vi "Sperre telebuf Minerva 27 Bytes (Sub VI).vi"(0 "Thruster rpms":dbl[](array[numeric]), 1 "manip1":u8, 2 "manip2":u8, 3 "manip3":u8, 4 "Pan_tilt":bool[](array[boolean]), 5 "error in":errorcluster, 6 "dim 1+2":u8, 7 "Lights_HMI":bool[](array[boolean]), 8 "dim 3+4":u8, 9 "Zoom":bool[](array[boolean]), 11 "Power":bool[](array[boolean]), 12 "camera":u8=2) -> (14 "telebuf":u8[](array[numeric]), 19 "error IO":errorcluster)   [LabVIEW 2014]
uses:
  <vilib>/imath/engines/lvmath2/RunTimeEngine/BuiltInFunctions/uint8/NIMS_uint8(int).vi
  <instcachedir>/0/NIMS_uint8(int)_9D6EF81F86254677BB00410F9E5C6A1D.lvgen/NIMS_uint8(int)_9D6EF81F86254677BB00410F9E5C6A1D_001.vi
  <vilib>/imath/engines/lvmath2/RunTimeEngine/BuiltInFunctions/round/NIMS_round(DBL-S).vi
  <vilib>/imath/engines/lvmath2/RunTimeEngine/BuiltInFunctions/uint8/NIMS_uint8(real).vi
  <instcachedir>/0/NIMS_uint8(real)_CAA419FBB1354DA296C59E18C46DECF0.lvgen/NIMS_uint8(real)_CAA419FBB1354DA296C59E18C46DECF0_000.vi
  <instcachedir>/0/NIMS_uint8(int)_9D6EF81F86254677BB00410F9E5C6A1D.lvgen/NIMS_uint8(int)_9D6EF81F86254677BB00410F9E5C6A1D_000.vi
  <vilib>/imath/engines/lvmath2/RunTimeEngine/IndexReplace/NIMS V(S)=S.vi
  <instcachedir>/0/NIMS V(S)=S_2D52C4EC15D8415E870AEE69FB516CCA.lvgen/NIMS V(S)=S_2D52C4EC15D8415E870AEE69FB516CCA_005.vi
  <vilib>/imathl/engines/lvmath/Functions/Error Handling/Create Error.vi
  <vilib>/imath/engines/lvmath2/RunTimeEngine/BuiltInFunctions/bitand/NIMS_bitand(SorS,SorS).vi
  <instcachedir>/0/NIMS V(S)=S_2D52C4EC15D8415E870AEE69FB516CCA.lvgen/NIMS V(S)=S_2D52C4EC15D8415E870AEE69FB516CCA_000.vi
  <vilib>/imath/engines/lvmath2/RunTimeEngine/ErrorHandling/NIMS_Create Error From Enums.vi
  <vilib>/imath/engines/lvmath2/RunTimeEngine/IndexRead/NIMS V(S).vi
  <instcachedir>/0/NIMS V(S)_0488751826AF41519A22953C041130DC.lvgen/NIMS V(S)_0488751826AF41519A22953C041130DC_000.vi
  <vilib>/imath/engines/lvmath2/RunTimeEngine/BuiltInFunctions/bitset/NIMS_bitset(RS,RS,RS).vi
  <vilib>/imath/engines/lvmath2/RunTimeEngine/BuiltInFunctions/bitget/NIMS_bitget(SorS,SorS).vi
  <vilib>/imath/engines/lvmath2/RunTimeEngine/RangeToken/NIMS_Range_R2 - Integer.vi
  <instcachedir>/0/NIMS_Range_R2 - Integer_2D1304BAF97744E0A293025746CBADFC.lvgen/NIMS_Range_R2 - Integer_2D1304BAF97744E0A293025746CBADFC_000.vi
  <vilib>/imath/engines/lvmath2/RunTimeEngine/CommandStatement/MC_CommandStatement_break.vi
  <vilib>/imath/engines/lvmath2/RunTimeEngine/BuiltInFunctions/double/NIMS_double.vi
  <instcachedir>/0/NIMS_double_34E32F64C2B04A25A042F4CA881A0A41.lvgen/NIMS_double_34E32F64C2B04A25A042F4CA881A0A41_002.vi
  <vilib>/imath/engines/lvmath2/RunTimeEngine/BuiltInFunctions/mod/NIMS_mod_no_size_check.vi
  <instcachedir>/0/NIMS_mod_no_size_check_5393E3382FD241D281EEB71DA286C65B.lvgen/NIMS_mod_no_size_check_5393E3382FD241D281EEB71DA286C65B_001.vi
  <vilib>/imath/engines/lvmath2/RunTimeEngine/NodeEndStatement/NIMS_NodeEndStatement_Output.vi
  <instcachedir>/0/NIMS_NodeEndStatement_Output_53EC0D466D134D7ABD903AC30B43404B.lvgen/NIMS_NodeEndStatement_Output_53EC0D466D134D7ABD903AC30B43404B_017.vi
  <vilib>/imath/engines/lvmath2/RunTimeEngine/ErrorHandling/NIMS_Finalize Error.vi
panel:
  in  "UHI camera":bool=TRUE
  in  "Turbo":bool=TRUE
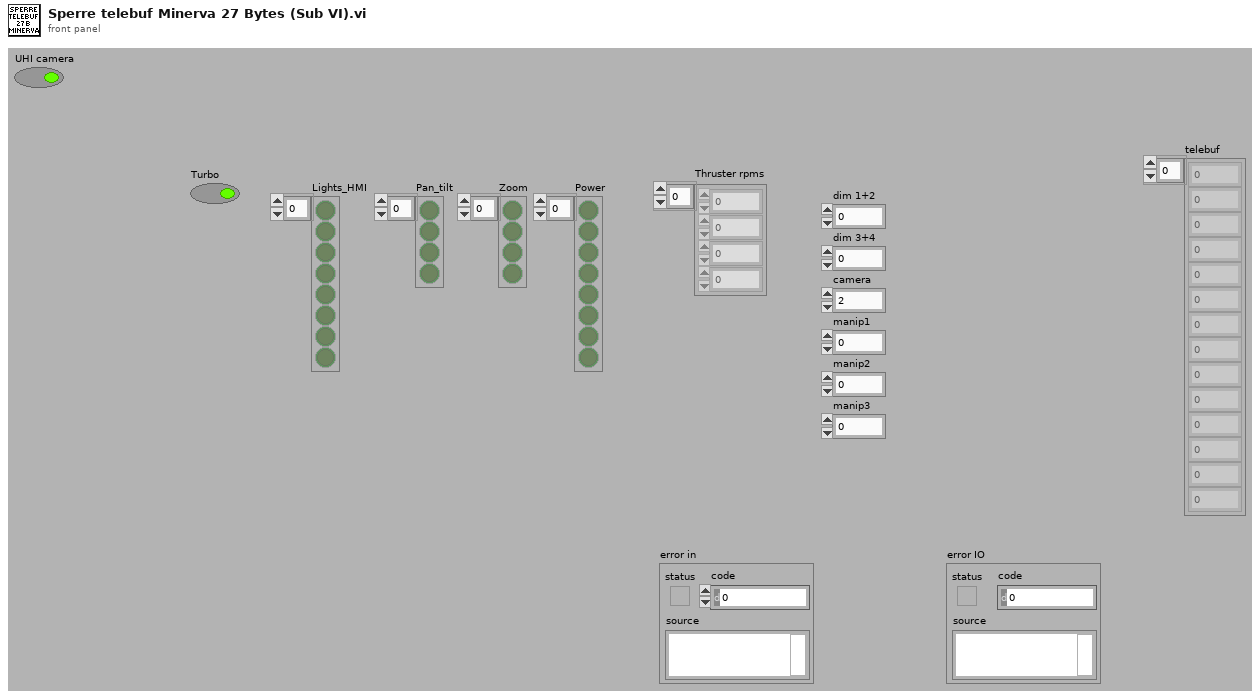
[diagram p1: front panel]
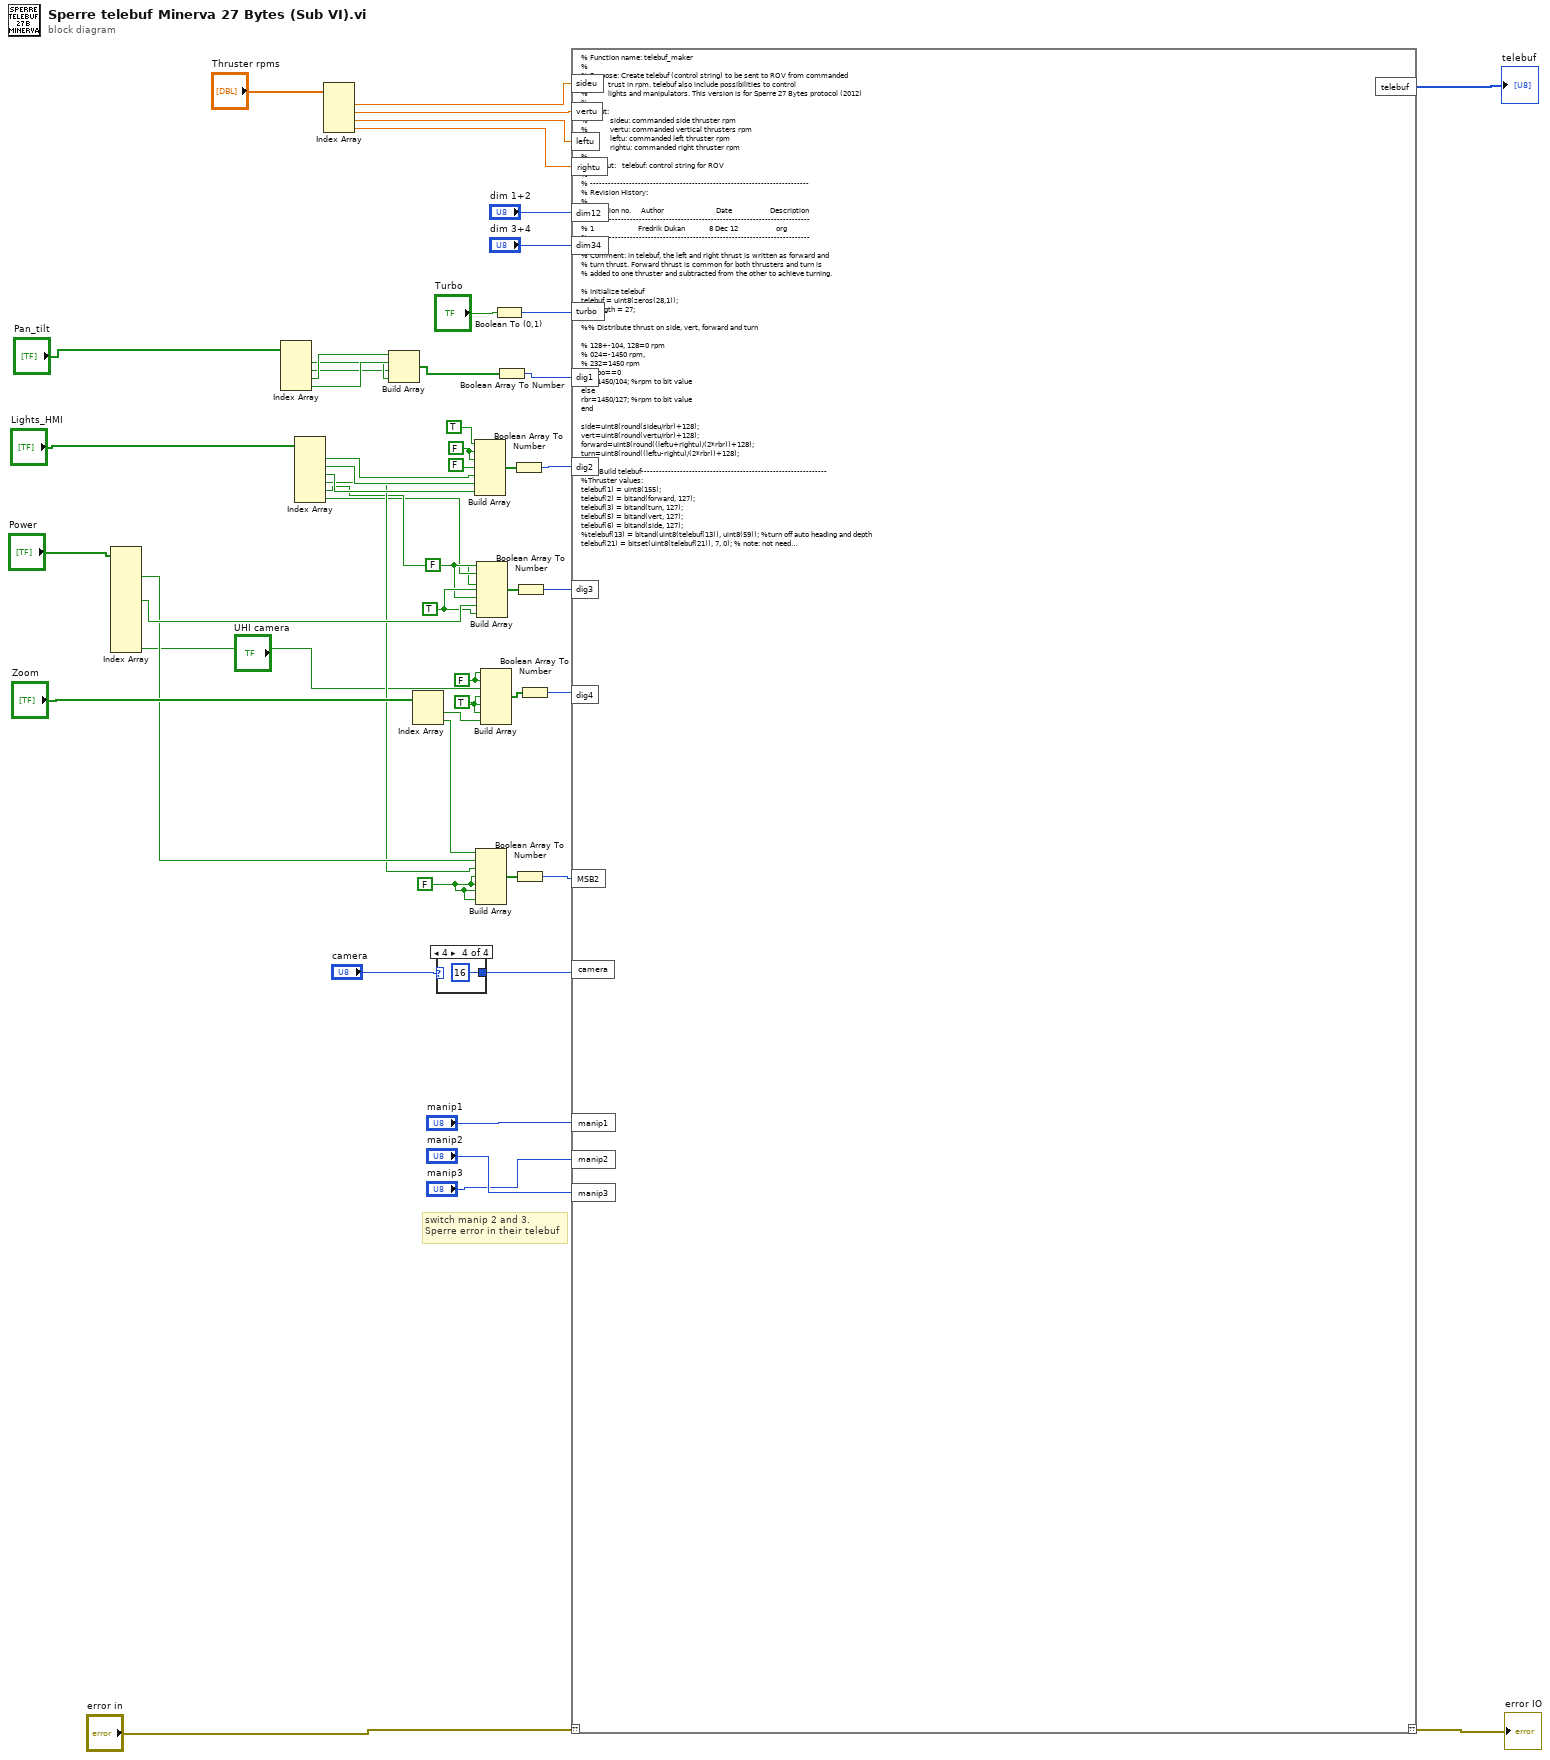
[diagram p0: block diagram]
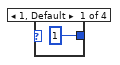
[diagram p2: hidden frame]
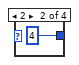
[diagram p3: hidden frame]
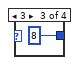
[diagram p4: hidden frame]
diagram:
  w18 = FALSE ("element")
  w22 = FALSE ("element")
  w4 = TRUE ("element")
  w2 = FALSE ("element")
  w29 = FALSE ("element")
  w5 = TRUE ("element")
  # "switch manip 2 and 3.\nSperre error in their telebuf"
  n1 = Index Array(array="Power") -> (element #2=w16:bool, element #5=w17:bool, element #11=w1:bool)  [unwired: 11 in, 8 out]
  n2 = Index Array(array="Pan_tilt") -> (element #1=w35:bool, element #2=w34:bool, element #3=w37:bool, element #4=w36:bool)  [unwired: 4 in]
  n3 = Index Array(array="Lights_HMI") -> (element #1=w13:bool, element #2=w12:bool, element #3=w11:bool, element #4=w10:bool, element #5=w9:bool, element #6=w3:bool)  [unwired: 6 in]
  n4 = Index Array(array="Thruster rpms") -> (element #1=w48:dbl, element #2=w47:dbl, element #3=w46:dbl, element #4=w45:dbl)  [unwired: 4 in]
  n5 = Build Array(w37, w36, w34, w35) -> (w33:bool[])
  n6 = Index Array(array="Zoom") -> (element #1=w6:bool, element #2=w23:bool)  [unwired: 2 in]
  n7 = case shown="4" "camera" {
    tunnel: [u8 1 u8 4 u8 8 u8 16] -> w21
    frame 1, Default {
    }
    frame 2 {
    }
    frame 3 {
    }
    frame 4 {
    }
  }
  n8 = Build Array(TRUE ("element"), w29, w29, FALSE ("element"), w13, w12, w11) -> (w31:bool[])
  n9 = Build Array(w23, w16, w10, w22, w22, w22, w22) -> (w25:bool[])
  n10 = Build Array(w9, w3, w2, w4, w2, w17, w4) -> (w27:bool[])
  n11 = Build Array(w18, w18, w1, w5, w5, w5, w6) -> (w41:bool[])
  n12 = Boolean To (0,1)(Boolean="Turbo") -> (0, 1=w14:i16)
  n13 = Boolean Array To Number(Boolean array=w33) -> (number=w32:u32)
  n14 = Boolean Array To Number(Boolean array=w31) -> (number=w30:u32)
  n15 = Boolean Array To Number(Boolean array=w25) -> (number=w24:u32)
  n16 = Boolean Array To Number(Boolean array=w27) -> (number=w26:u32)
  n17 = Boolean Array To Number(Boolean array=w41) -> (number=w40:u32)
  n18 = mathscript code="% Function name: telebuf_maker\n%\n% Purpose: Create telebuf (control string) to be sent to ROV from commanded\n%          trust in rpm. telebuf also include possibilities to control\n%          lights and manipulators. This version is for Sperre 27 Bytes protocol (2012)\n%\n% Input:  \n%           sideu: commanded side thruster rpm\n%           vertu: commanded vertical thrusters rpm\n%           leftu: commanded left thruster rpm\n%           rightu: commanded right thruster rpm\n%\n% Output:   telebuf: control string for ROV\n%\n% -------------------------------------------------------------------------\n% Revision History:\n%\n% Revision no.     Author                          Date                   Description\n%--------------------------------------------------------------------------\n% 1                      Fredrik Dukan            8 Dec 12                   org  \n%--------------------------------------------------------------------------\n\n% Comment: in telebuf, the left and right thrust is written as forward and\n% turn thrust. Forward thrust is common for both thrusters and turn is \n% added to one thruster and subtracted from the other to achieve turning.\n\n% Initialize telebuf\ntelebuf = uint8(zeros(28,1));\ntelelength = 27;\n\n%% Distribute thrust on side, vert, forward and turn\n\n% 128+-104, 128=0 rpm\n% 024=-1450 rpm,\n% 232=1450 rpm\nif turbo==0\nrbr=1450/104; %rpm to bit value\nelse\nrbr=1450/127; %rpm to bit value\nend\n\nside=uint8(round(sideu/rbr)+128);\nvert=uint8(round(vertu/rbr)+128);\nforward=uint8(round((leftu+rightu)/(2*rbr))+128);\nturn=uint8(round((leftu-rightu)/(2*rbr))+128);\n\n%%  Build telebuf--------------------------------------------------------------\n%Thruster values:\ntelebuf(1) = uint8(155);\ntelebuf(2) = bitand(forward, 127);\ntelebuf(3) = bitand(turn, 127);\ntelebuf(5) = bitand(vert, 127);\ntelebuf(6) = bitand(side, 127);\n%telebuf(13) = bitand(uint8(telebuf(13)), uint8(59)); %turn off auto heading and depth\ntelebuf(21) = bitset(uint8(telebuf(21)), 7, 0); % note: not needed in matlab\ntelebuf(21) = bitset(uint8(telebuf(21)), 7, bitget(forward, 8)); %0x40\ntelebuf(21) = bitset(uint8(telebuf(21)), 6, 0); % note: not needed in matlab\ntelebuf(21) = bitset(uint8(telebuf(21)), 6, bitget(turn, 8)); %0x20\ntelebuf(21) = bitset(uint8(telebuf(21)), 5, 1); % note: not needed in matlab\ntelebuf(21) = bitset(uint8(telebuf(21)), 4, 0); % note: not needed in matlab\ntelebuf(21) = bitset(uint8(telebuf(21)), 4, bitget(vert, 8));  %0x08\ntelebuf(21) = bitset(uint8(telebuf(21)), 3, 0); % note: not needed in matlab\ntelebuf(21) = bitset(uint8(telebuf(21)), 3, bitget(side, 8)); %0x04\ntelebuf(21) = bitset(uint8(telebuf(21)), 2, 1); % note: not needed in matlab\n%Misc switches -------------------------------------------------------------------\ntelebuf(9) = dim12;            %Dimm1 (byte no 8)\ntelebuf(10) = dim12;          %Dimm2 (byte no 9)\ntelebuf(11) = dim34;          %Dimm3 (byte no 10)\ntelebuf(12) = uint8(64);      %Ext_thr (byte no 11)  set to dummy value\n%telebuf(13) = dim34;        %fwd pot (byte no 12)\ntelebuf(14) =dim34;            %Dimm4 (byte no 13)\n%telebuf(15) =uint8(0);       %Spare (byte no 14)  set to dummy value\n%telebuf(16) =uint8(0);       %Spare (byte no 15)  set to dummy value\ntelebuf(17) =dig1;                %Dig1 (byte no 16) \ntelebuf(18) =dig2;                %Dig2 (byte no 17) \ntelebuf(19) =dig3;                %Dig3 (byte no 18) \ntelebuf(20) =dig4;                %Dig4 (byte no 19) \n\ntelebuf(22) =MSB2;               %MSBs (byte no 21) \ntelebuf(23) =camera;            %Camera select (byte no 22) \n\ntelebuf(24) = manip1;         %Manip1 (byte no 23) \ntelebuf(25) = manip2;         %Manip2 (byte no 24) \ntelebuf(26) = manip3;         %Manip3 (byte no 25) \n\n%checksums:-----------------------------------------------------------------------\nchk = uint8(0);\n\nfor i = 1:telelength - 1\n    chk = chk + telebuf(i);\nend\nchk1 = double(chk);\ncheck1 = bitand(uint8(floor(chk1/256)), 127);\ncheck2 = bitand(mod(chk, 256) , 127);\ntelebuf(27) = check1;       %checksum (byte no 26) \ntelebuf(28) = check2;       %checksum (byte no 27)"("??"="error in", "sideu"=w48, "vertu"=w47, "leftu"=w46, "rightu"=w45, "dim12"="dim 1+2", "dim34"="dim 3+4", "manip1"="manip1", "manip2"="manip3", "manip3"="manip2", "dig2"=w30, "dig3"=w26, "dig4"=w40, "dig1"=w32, "MSB2"=w24, "camera"=w21, "turbo"=w14) -> ("??"=→"error IO":errorcluster, "telebuf"=→"telebuf":u8[])
